vi "AutoAlign.vi"() -> ()   [LabVIEW 2019]
uses:
  Framework/Robot Global Data.vi
panel:
  in  "NoWait":bool
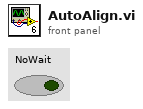
[diagram p1: front panel]
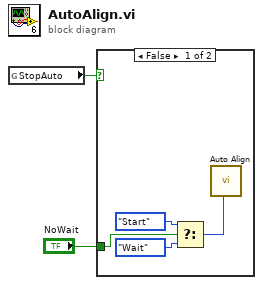
[diagram p0: block diagram]
diagram:
  n1 = global read "Robot Global Data.vi" "StopAuto"() -> (w1:bool)
  n2 = case shown="False" w1 {
    tunnel: "NoWait" -> [w4 _]
    frame False {
      n3 = Select(t=enum16{"Start", "Wait"}."Start" ("Synchronization"), s=w4, f=enum16{"Start", "Wait"}."Wait" ("Synchronization")) -> (s? t:f=w3:enum16{"Start", "Wait"})
      n4 = call "Auto Align.vi"("Synchronication"=w3) -> ()  [unwired: 10 in, 1 out]
    }
    frame True {
    }
  }
